vi "move_last_to_first.vi"(11 "Input array":dbl[](array[numeric])) -> (3 "Output Array":dbl[](array[numeric]))   [LabVIEW 2018]
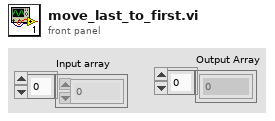
[diagram p1: front panel]
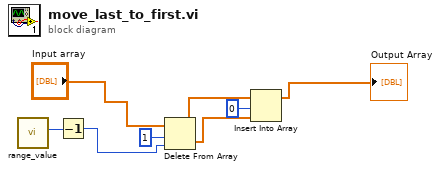
[diagram p0: block diagram]
diagram:
  n1 = call "range_value.vi"() -> ("NumBins"=w8:i32)  [unwired: 10 in, 1 out]
  n2 = Decrement(x=w8) -> (x-1=w5:i32)
  n3 = Delete From Array(array="Input array", length=1, index=w5) -> (deleted portion=w4:dbl[], array with subset deleted=w3:dbl[])
  n4 = Insert Into Array(array=w3, index=0, new element=w4) -> (→"Output Array":dbl[])
